vi "Base10 To Base36.vi"(2 "Base 10":u64) -> (0 "Base36":string, 1 "length":i32)   [LabVIEW 2016]
panel:
  out "size(s)":i32
  out "Base 10":u64 format="%#_4g"
  # "Letter o has been replaced with -\nNumber 0 has been replaced with *"
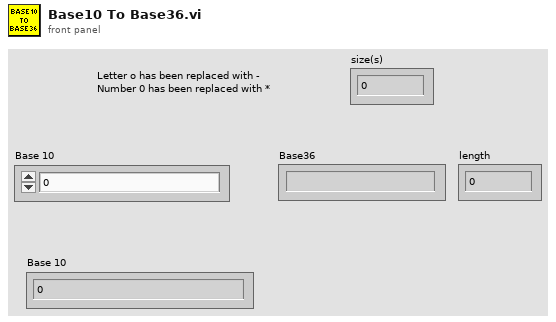
[diagram p1: front panel]
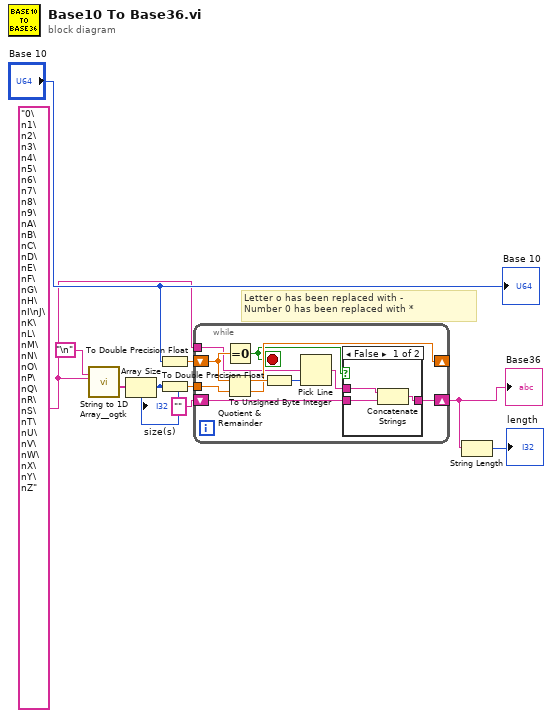
[diagram p0: block diagram]
diagram:
  w7 = "0\n1\n2\n3\n4\n5\n6\n7\n8\n9\nA\nB\nC\nD\nE\nF\nG\nH\nI\nJ\nK\nL\nM\nN\nO\nP\nQ\nR\nS\nT\nU\nV\nW\nX\nY\nZ" ("multi-line string")
  # "Letter o has been replaced with -\nNumber 0 has been replaced with *"
  n1 = call <userlib>:"String to 1D Array__ogtk.vi"("delimiter (Tab)"="\n", "string"=w7) -> ("Array of Strings"=w6:string[])  [unwired: 9 in]
  n2 = Array Size(array=w6) -> (size(s)=w4:i32)
  "size(s)" <- w4
  n3 = To Double Precision Float(number="Base 10") -> (double precision float=w9:dbl)
  n4 = To Double Precision Float(number=w4) -> (double precision float=w3:dbl)
  n5 = while {
    shift-right: [w18] -> _
    shift-left: w9 -> [w20]
    tunnel: w7 -> [w15]
    tunnel: w3 -> [w14]
    shift-right: [w13] -> w1
    shift-left: "" -> [w12]
    stop <- w17 stop-if-true
    n6 = Equal To 0?(x=w20) -> (x = 0?=w17:bool)
    n7 = Quotient & Remainder(x=w20, y=w14) -> (x-y*floor(x/y)=w19:dbl, floor(x/y)=w18:dbl)
    n8 = To Unsigned Byte Integer(number=w19) -> (unsigned 8bit integer=w16:u8)
    n9 = Pick Line(multi-line string=w15, line index=w16) -> (output string=w11:string)  [unwired: 1 in]
    n10 = case shown="False" w17 {
      tunnel: [w22 w24] -> w13
      tunnel: w12 -> [w23 w24]
      tunnel: w11 -> [w21 _]
      frame False {
        n11 = Concatenate Strings(w21, w23) -> (w22:string)
      }
      frame True {
      }
    }
  }
  "Base36" <- w1
  n12 = String Length(string=w1) -> (length=→"length":i32)
  "Base 10" <- "Base 10"
